vi "Host Matsya 6000.vi"(6 "Channel Data":cluster{"AI":T1, "DI":T5, "DO":T5, "Async":T8}={"AI"={"Interface"="AIO", "Interface Data"={"Command"="Configure", "SubCmd"="AI", "Data"=[{"Channel"="Mod2/ai0", "Min Value"=-5.0, "Max Value"=5.0, "Type"="Voltage", "Terminal Configure"=10083, "Dynamic"=0, "Dyn Type"="", "Data"=[], "File Name"="", "Column"=0, "Frequency"=0.0}, {"Channel"="Mod2/ai1", "Min Value"=-5.0, "Max Value"=5.0, "Type"="Voltage", "Terminal Configure"=10083, "Dynamic"=0, "Dyn Type"="", "Data"=[], "File Name"="", "Column"=0, "Frequency"=0.0}, {"Channel"="Mod2/ai2", "Min Value"=-5.0, "Max Value"=5.0, "Type"="Voltage", "Terminal Configure"=10083, "Dynamic"=0, "Dyn Type"="", "Data"=[], "File Name"="", "Column"=0, "Frequency"=0.0}, {"Channel"="Mod2/ai3", "Min Value"=-5.0, "Max Value"=5.0, "Type"="Voltage", "Terminal Configure"=10083, "Dynamic"=0, "Dyn Type"="", "Data"=[], "File Name"="", "Column"=0, "Frequency"=0.0}, {"Channel"="Mod2/ai4", "Min Value"=-5.0, "Max Value"=5.0, "Type"="Voltage", "Terminal Configure"=10083, "Dynamic"=0, "Dyn Type"="", "Data"=[], "File Name"="", "Column"=0, "Frequency"=0.0}, {"Channel"="Mod2/ai5", "Min Value"=-5.0, "Max Value"=5.0, "Type"="Voltage", "Terminal Configure"=10083, "Dynamic"=0, "Dyn Type"="", "Data"=[], "File Name"="", "Column"=0, "Frequency"=0.0}, {"Channel"="Mod2/ai6", "Min Value"=-5.0, "Max Value"=5.0, "Type"="Voltage", "Terminal Configure"=10083, "Dynamic"=0, "Dyn Type"="", "Data"=[], "File Name"="", "Column"=0, "Frequency"=0.0}, {"Channel"="Mod2/ai7", "Min Value"=-5.0, "Max Value"=5.0, "Type"="Voltage", "Terminal Configure"=10083, "Dynamic"=0, "Dyn Type"="", "Data"=[], "File Name"="", "Column"=0, "Frequency"=0.0}, {"Channel"="Mod2/ai8", "Min Value"=-5.0, "Max Value"=5.0, "Type"="Voltage", "Terminal Configure"=10083, "Dynamic"=0, "Dyn Type"="", "Data"=[], "File Name"="", "Column"=0, "Frequency"=0.0}, {"Channel"="Mod2/ai9", "Min Value"=-5.0, "Max Value"=5.0, "Type"="Voltage", "Terminal Configure"=10083, "Dynamic"=0, "Dyn Type"="", "Data"=[], "File Name"="", "Column"=0, "Frequency"=0.0}, {"Channel"="Mod2/ai10", "Min Value"=-5.0, "Max Value"=5.0, "Type"="Voltage", "Terminal Configure"=10083, "Dynamic"=0, "Dyn Type"="", "Data"=[], "File Name"="", "Column"=0, "Frequency"=0.0}, {"Channel"="Mod2/ai11", "Min Value"=-5.0, "Max Value"=5.0, "Type"="Voltage", "Terminal Configure"=10083, "Dynamic"=0, "Dyn Type"="", "Data"=[], "File Name"="", "Column"=0, "Frequency"=0.0}, {"Channel"="Mod2/ai12", "Min Value"=-5.0, "Max Value"=5.0, "Type"="Voltage", "Terminal Configure"=10083, "Dynamic"=0, "Dyn Type"="", "Data"=[], "File Name"="", "Column"=0, "Frequency"=0.0}, {"Channel"="Mod2/ai13", "Min Value"=-5.0, "Max Value"=5.0, "Type"="Voltage", "Terminal Configure"=10083, "Dynamic"=0, "Dyn Type"="", "Data"=[], "File Name"="", "Column"=0, "Frequency"=0.0}, {"Channel"="Mod2/ai14", "Min Value"=-5.0, "Max Value"=5.0, "Type"="Voltage", "Terminal Configure"=10083, "Dynamic"=0, "Dyn Type"="", "Data"=[], "File Name"="", "Column"=0, "Frequency"=0.0}, {"Channel"="Mod2/ai15", "Min Value"=-5.0, "Max Value"=5.0, "Type"="Voltage", "Terminal Configure"=10083, "Dynamic"=0, "Dyn Type"="", "Data"=[], "File Name"="", "Column"=0, "Frequency"=0.0}, {"Channel"="Mod2/ai16", "Min Value"=-5.0, "Max Value"=5.0, "Type"="Voltage", "Terminal Configure"=10083, "Dynamic"=0, "Dyn Type"="", "Data"=[], "File Name"="", "Column"=0, "Frequency"=0.0}, {"Channel"="Mod2/ai17", "Min Value"=-5.0, "Max Value"=5.0, "Type"="Voltage", "Terminal Configure"=10083, "Dynamic"=0, "Dyn Type"="", "Data"=[], "File Name"="", "Column"=0, "Frequency"=0.0}, {"Channel"="Mod2/ai18", "Min Value"=-5.0, "Max Value"=5.0, "Type"="Voltage", "Terminal Configure"=10083, "Dynamic"=0, "Dyn Type"="", "Data"=[], "File Name"="", "Column"=0, "Frequency"=0.0}, {"Channel"="Mod2/ai19", "Min Value"=-5.0, "Max Value"=5.0, "Type"="Voltage", "Terminal Configure"=10083, "Dynamic"=0, "Dyn Type"="", "Data"=[], "File Name"="", "Column"=0, "Frequency"=0.0}, {"Channel"="Mod2/ai20", "Min Value"=-5.0, "Max Value"=5.0, "Type"="Voltage", "Terminal Configure"=10083, "Dynamic"=0, "Dyn Type"="", "Data"=[], "File Name"="", "Column"=0, "Frequency"=0.0}, {"Channel"="Mod2/ai21", "Min Value"=-5.0, "Max Value"=5.0, "Type"="Voltage", "Terminal Configure"=10083, "Dynamic"=0, "Dyn Type"="", "Data"=[], "File Name"="", "Column"=0, "Frequency"=0.0}, {"Channel"="Mod2/ai22", "Min Value"=-5.0, "Max Value"=5.0, "Type"="Voltage", "Terminal Configure"=10083, "Dynamic"=0, "Dyn Type"="", "Data"=[], "File Name"="", "Column"=0, "Frequency"=0.0}, {"Channel"="Mod2/ai23", "Min Value"=-5.0, "Max Value"=5.0, "Type"="Voltage", "Terminal Configure"=10083, "Dynamic"=0, "Dyn Type"="", "Data"=[], "File Name"="", "Column"=0, "Frequency"=0.0}, {"Channel"="Mod2/ai24", "Min Value"=-5.0, "Max Value"=5.0, "Type"="Voltage", "Terminal Configure"=10083, "Dynamic"=0, "Dyn Type"="", "Data"=[], "File Name"="", "Column"=0, "Frequency"=0.0}, {"Channel"="Mod2/ai25", "Min Value"=-5.0, "Max Value"=5.0, "Type"="Voltage", "Terminal Configure"=10083, "Dynamic"=0, "Dyn Type"="", "Data"=[], "File Name"="", "Column"=0, "Frequency"=0.0}, {"Channel"="Mod2/ai26", "Min Value"=-5.0, "Max Value"=5.0, "Type"="Voltage", "Terminal Configure"=10083, "Dynamic"=0, "Dyn Type"="", "Data"=[], "File Name"="", "Column"=0, "Frequency"=0.0}, {"Channel"="Mod2/ai27", "Min Value"=-5.0, "Max Value"=5.0, "Type"="Voltage", "Terminal Configure"=10083, "Dynamic"=0, "Dyn Type"="", "Data"=[], "File Name"="", "Column"=0, "Frequency"=0.0}, {"Channel"="Mod2/ai28", "Min Value"=-5.0, "Max Value"=5.0, "Type"="Voltage", "Terminal Configure"=10083, "Dynamic"=0, "Dyn Type"="", "Data"=[], "File Name"="", "Column"=0, "Frequency"=0.0}, {"Channel"="Mod2/ai29", "Min Value"=-5.0, "Max Value"=5.0, "Type"="Voltage", "Terminal Configure"=10083, "Dynamic"=0, "Dyn Type"="", "Data"=[], "File Name"="", "Column"=0, "Frequency"=0.0}, {"Channel"="Mod2/ai30", "Min Value"=-5.0, "Max Value"=5.0, "Type"="Voltage", "Terminal Configure"=10083, "Dynamic"=0, "Dyn Type"="", "Data"=[], "File Name"="", "Column"=0, "Frequency"=0.0}, {"Channel"="Mod2/ai31", "Min Value"=-5.0, "Max Value"=5.0, "Type"="Voltage", "Terminal Configure"=65535, "Dynamic"=0, "Dyn Type"="", "Data"=[], "File Name"="", "Column"=0, "Frequency"=0.0}], "Timing"={"samples per channel"=4, "sample mode"=10123, "rate"=2.0}}}, "DI"={"Interface"="DIO", "Interface Data"={"Command"="Configure", "SubCmd"="DI", "Frequency"=500, "Data"=[{"Channel"="Mod3/port0/line0", "Data"=[0], "Identification Name"=""}, {"Channel"="Mod3/port0/line1", "Data"=[0], "Identification Name"=""}, {"Channel"="Mod3/port0/line2", "Data"=[0], "Identification Name"=""}, {"Channel"="Mod3/port0/line3", "Data"=[0], "Identification Name"=""}, {"Channel"="Mod3/port0/line4", "Data"=[0], "Identification Name"=""}, {"Channel"="Mod3/port0/line5", "Data"=[0], "Identification Name"=""}, {"Channel"="Mod3/port0/line6", "Data"=[0], "Identification Name"=""}, {"Channel"="Mod3/port0/line7", "Data"=[0], "Identification Name"=""}, {"Channel"="Mod3/port0/line8", "Data"=[0], "Identification Name"=""}, {"Channel"="Mod3/port0/line9", "Data"=[0], "Identification Name"=""}, {"Channel"="Mod3/port0/line10", "Data"=[0], "Identification Name"=""}, {"Channel"="Mod3/port0/line11", "Data"=[0], "Identification Name"=""}, {"Channel"="Mod3/port0/line12", "Data"=[0], "Identification Name"=""}, {"Channel"="Mod3/port0/line13", "Data"=[0], "Identification Name"=""}, {"Channel"="Mod3/port0/line14", "Data"=[0], "Identification Name"=""}, {"Channel"="Mod3/port0/line15", "Data"=[0], "Identification Name"=""}, {"Channel"="Mod3/port0/line16", "Data"=[0], "Identification Name"=""}, {"Channel"="Mod3/port0/line17", "Data"=[0], "Identification Name"=""}, {"Channel"="Mod3/port0/line18", "Data"=[0], "Identification Name"=""}, {"Channel"="Mod3/port0/line19", "Data"=[0], "Identification Name"=""}, {"Channel"="Mod3/port0/line20", "Data"=[0], "Identification Name"=""}, {"Channel"="Mod3/port0/line21", "Data"=[0], "Identification Name"=""}, {"Channel"="Mod3/port0/line22", "Data"=[0], "Identification Name"=""}, {"Channel"="Mod3/port0/line23", "Data"=[0], "Identification Name"=""}, {"Channel"="Mod3/port0/line24", "Data"=[0], "Identification Name"=""}, {"Channel"="Mod3/port0/line25", "Data"=[0], "Identification Name"=""}, {"Channel"="Mod3/port0/line26", "Data"=[0], "Identification Name"=""}, {"Channel"="Mod3/port0/line27", "Data"=[0], "Identification Name"=""}, {"Channel"="Mod3/port0/line28", "Data"=[0], "Identification Name"=""}, {"Channel"="Mod3/port0/line29", "Data"=[0], "Identification Name"=""}, {"Channel"="Mod3/port0/line30", "Data"=[0], "Identification Name"=""}, {"Channel"="Mod3/port0/line31", "Data"=[0], "Identification Name"=""}, {"Channel"="Mod4/port0/line0", "Data"=[0], "Identification Name"=""}, {"Channel"="Mod4/port0/line1", "Data"=[0], "Identification Name"=""}, {"Channel"="Mod4/port0/line2", "Data"=[0], "Identification Name"=""}, {"Channel"="Mod4/port0/line3", "Data"=[0], "Identification Name"=""}, {"Channel"="Mod4/port0/line4", "Data"=[0], "Identification Name"=""}, {"Channel"="Mod4/port0/line5", "Data"=[0], "Identification Name"=""}, {"Channel"="Mod4/port0/line6", "Data"=[0], "Identification Name"=""}, {"Channel"="Mod4/port0/line7", "Data"=[0], "Identification Name"=""}, {"Channel"="Mod4/port0/line8", "Data"=[0], "Identification Name"=""}, {"Channel"="Mod4/port0/line9", "Data"=[0], "Identification Name"=""}, {"Channel"="Mod4/port0/line10", "Data"=[0], "Identification Name"=""}, {"Channel"="Mod4/port0/line11", "Data"=[0], "Identification Name"=""}, {"Channel"="Mod4/port0/line12", "Data"=[0], "Identification Name"=""}, {"Channel"="Mod4/port0/line13", "Data"=[0], "Identification Name"=""}, {"Channel"="Mod4/port0/line14", "Data"=[0], "Identification Name"=""}, {"Channel"="Mod4/port0/line15", "Data"=[0], "Identification Name"=""}, {"Channel"="Mod4/port0/line16", "Data"=[0], "Identification Name"=""}, {"Channel"="Mod4/port0/line17", "Data"=[0], "Identification Name"=""}, {"Channel"="Mod4/port0/line18", "Data"=[0], "Identification Name"=""}, {"Channel"="Mod4/port0/line19", "Data"=[0], "Identification Name"=""}, {"Channel"="Mod4/port0/line20", "Data"=[0], "Identification Name"=""}, {"Channel"="Mod4/port0/line21", "Data"=[0], "Identification Name"=""}, {"Channel"="Mod4/port0/line22", "Data"=[0], "Identification Name"=""}, {"Channel"="Mod4/port0/line23", "Data"=[0], "Identification Name"=""}, {"Channel"="Mod4/port0/line24", "Data"=[0], "Identification Name"=""}, {"Channel"="Mod4/port0/line25", "Data"=[0], "Identification Name"=""}, {"Channel"="Mod4/port0/line26", "Data"=[0], "Identification Name"=""}, {"Channel"="Mod4/port0/line27", "Data"=[0], "Identification Name"=""}, {"Channel"="Mod4/port0/line28", "Data"=[0], "Identification Name"=""}, {"Channel"="Mod4/port0/line29", "Data"=[0], "Identification Name"=""}, {"Channel"="Mod4/port0/line30", "Data"=[0], "Identification Name"=""}, {"Channel"="Mod4/port0/line31", "Data"=[0], "Identification Name"=""}]}}, "DO"={"Interface"="DIO", "Interface Data"={"Command"="Configure", "SubCmd"="DO", "Frequency"=500, "Data"=[{"Channel"="Mod1/port0/line0", "Data"=[0], "Identification Name"=""}, {"Channel"="Mod1/port0/line1", "Data"=[0], "Identification Name"=""}, {"Channel"="Mod1/port0/line2", "Data"=[0], "Identification Name"=""}, {"Channel"="Mod1/port0/line3", "Data"=[0], "Identification Name"=""}, {"Channel"="Mod1/port0/line4", "Data"=[0], "Identification Name"=""}, {"Channel"="Mod1/port0/line5", "Data"=[0], "Identification Name"=""}, {"Channel"="Mod1/port0/line6", "Data"=[0], "Identification Name"=""}, {"Channel"="Mod1/port0/line7", "Data"=[0], "Identification Name"=""}, {"Channel"="Mod1/port0/line8", "Data"=[0], "Identification Name"=""}, {"Channel"="Mod1/port0/line9", "Data"=[0], "Identification Name"=""}, {"Channel"="Mod1/port0/line10", "Data"=[0], "Identification Name"=""}, {"Channel"="Mod1/port0/line11", "Data"=[0], "Identification Name"=""}, {"Channel"="Mod1/port0/line12", "Data"=[0], "Identification Name"=""}, {"Channel"="Mod1/port0/line13", "Data"=[0], "Identification Name"=""}, {"Channel"="Mod1/port0/line14", "Data"=[0], "Identification Name"=""}, {"Channel"="Mod1/port0/line15", "Data"=[0], "Identification Name"=""}, {"Channel"="Mod1/port0/line16", "Data"=[0], "Identification Name"=""}, {"Channel"="Mod1/port0/line17", "Data"=[0], "Identification Name"=""}, {"Channel"="Mod1/port0/line18", "Data"=[0], "Identification Name"=""}, {"Channel"="Mod1/port0/line19", "Data"=[0], "Identification Name"=""}, {"Channel"="Mod1/port0/line20", "Data"=[0], "Identification Name"=""}, {"Channel"="Mod1/port0/line21", "Data"=[0], "Identification Name"=""}, {"Channel"="Mod1/port0/line22", "Data"=[0], "Identification Name"=""}, {"Channel"="Mod1/port0/line23", "Data"=[0], "Identification Name"=""}, {"Channel"="Mod1/port0/line24", "Data"=[0], "Identification Name"=""}, {"Channel"="Mod1/port0/line25", "Data"=[0], "Identification Name"=""}, {"Channel"="Mod1/port0/line26", "Data"=[0], "Identification Name"=""}, {"Channel"="Mod1/port0/line27", "Data"=[0], "Identification Name"=""}, {"Channel"="Mod1/port0/line28", "Data"=[0], "Identification Name"=""}, {"Channel"="Mod1/port0/line29", "Data"=[0], "Identification Name"=""}, {"Channel"="Mod1/port0/line30", "Data"=[0], "Identification Name"=""}, {"Channel"="Mod1/port0/line31", "Data"=[0], "Identification Name"=""}]}}, "Async"={"Interface"="Async", "Interface Data"={"Command"="Configure", "SubCmd"="Async", "Data"=[{"Port"="com10", "Minor Frame Freq"=200, "Minor Frame Count"=1, "Frame Info"=[{"Frame ID"=1, "Message Info"=[{"Message"=[1], "Message Name"="m1"}]}], "Sensor Type"=0, "OIM Address"=0}]}}} {"Async"."Interface Data"."Data"."Minor Frame Count" min=5 max=8 step=1; "AI"."Interface Data"."Timing"."sample mode" items=["Finite Samples"=10178, "Continuous Samples"=10123, "Hardware Timed Single Point"=12522]}, 11 "address":string="192.168.81.153") -> ()   [LabVIEW 2021]
uses:
  Main Engine/Controls/Main Engine CPU Info.ctl
  Host/Controls/Host Data Cluster.ctl
  Async Serial/Controls/Async Update Cluster.ctl
  Async Serial/Controls/Async Message Info Cluster.ctl
  Analog Output/Controls/AO Timing Cluster.ctl
  Analog Output/Controls/AO Channel Configuration Cluster.ctl
  Analog Output/Controls/AO Interface Data Cluster.ctl
  Analog Output/Controls/AO JSON Data Cluster.ctl
  Digital Output/SubVIs/Digital Dynamic Cluster.ctl
  Digital Output/Controls/DIO Interface Data.ctl
  Digital Output/Controls/DIO Configuration cluster.ctl
  Async Serial/Controls/Async Frame Info Cluster.ctl
  Async Serial/Controls/Async Serial Configuration Cluster.ctl
  Host/Async Interface Data Cluster.ctl
  Host/Async JSON Cluster.ctl
panel:
  out "error out 3":errorcluster
  out "error out 2":errorcluster
  out "Data Out":T13
  out "Stop":bool
  out "error out":errorcluster
  in  "Tab Control":T15(tab)
  in  "Send DIO Update":bool
  in  "DO Data":cluster{"Channel":string[], "Data":u8[]}={"Channel"=["Mod2/port1/line0", "Mod2/port1/line1", "Mod2/port1/line2", "Mod2/port1/line3"], "Data"=[0, 0, 0, 0]}
  in  "Send Async Update":bool
  in  "Serial Data":T16[](array[typedef])
  in  "Async Stop":string="{\"Interface\":\"Async\",\"Interface Data\":{\"Command\":\"Stop\",\"SubCmd\":\"Async\",\"Data\":[\"com2\"]}}"
  in  "Send Async Stop":bool
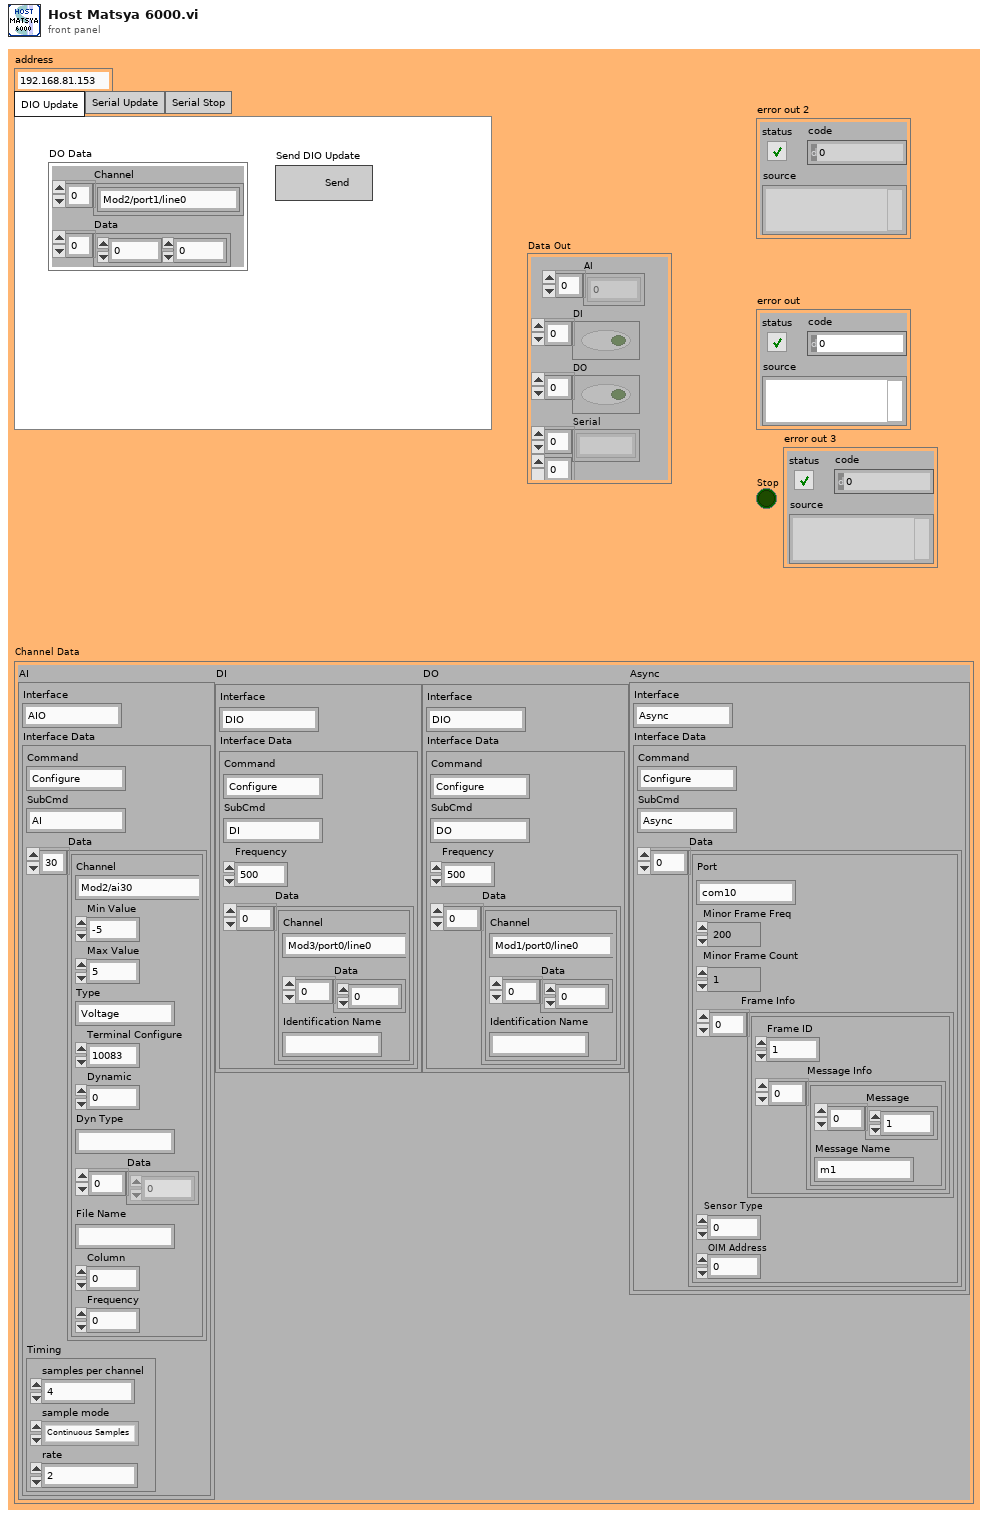
[diagram p1: front panel]
types:
  T1 = typedef "AO JSON Data Cluster.ctl" = cluster{"Interface":string, "Interface Data":T2}
  T2 = typedef "AO Interface Data Cluster.ctl" = cluster{"Command":string, "SubCmd":string, "Data":T3[], "Timing":T4}
  T3 = typedef "AO Channel Configuration Cluster.ctl" = cluster{"Channel":string, "Min Value":dbl, "Max Value":dbl, "Type":string, "Terminal Configure":u16, "Dynamic":u8, "Dyn Type":string, "Data":dbl[], "File Name":string, "Column":i32, "Frequency":dbl}
  T4 = typedef "AO Timing Cluster.ctl" = cluster{"samples per channel":i32, "sample mode":i32, "rate":dbl}
  T5 = typedef "DIO Configuration cluster.ctl" = cluster{"Interface":string, "Interface Data":T6}
  T6 = typedef "DIO Interface Data.ctl" = cluster{"Command":string, "SubCmd":string, "Frequency":u16, "Data":T7[]}
  T7 = typedef "Digital Dynamic Cluster.ctl" = cluster{"Channel":string, "Data":u8[], "Identification Name":string}
  T8 = typedef "Async JSON Cluster.ctl" = cluster{"Interface":string, "Interface Data":T9}
  T9 = typedef "Async Interface Data Cluster.ctl" = cluster{"Command":string, "SubCmd":string, "Data":T10[]}
  T10 = typedef "Async Serial Configuration Cluster.ctl" = cluster{"Port":string, "Minor Frame Freq":u16, "Minor Frame Count":u16, "Frame Info":T11[], "Sensor Type":u16, "OIM Address":u16}
  T11 = typedef "Async Frame Info Cluster.ctl" = cluster{"Frame ID":u16, "Message Info":T12[]}
  T12 = typedef "Async Message Info Cluster.ctl" = cluster{"Message":u8[], "Message Name":string}
  T13 = typedef "Host Data Cluster.ctl" = cluster{"AI":dbl[], "DI":bool[], "DO":bool[], "Serial":string[][], "CPU":T14, "Stop":bool, "DO Channel":string[]}
  T14 = typedef "Main Engine CPU Info.ctl" = cluster{"Total Load":u32[], "Interrupt Load":u32[], "Total Physical":dbl, "Free Physical":dbl, "Primary Disk Capacity":dbl, "Primary Disk Free":dbl}
  T15 = enum32{"DIO Update", "DIO stop", "Serial Update", "Serial Stop"}
  T16 = typedef "Async Update Cluster.ctl" = cluster{"Port":string, "Message Info":T12[]}
  T17 = enum16{"Initialize", "Read", "Update DO", "Update Serial", "Exit"}
  T18 = enum16{"big-endian, network order", "native, host order", "little-endian"}
  T19 = typedef "RT Data's.ctl" = cluster{"RT HW Info":T20, "DO Info":T24}
  T20 = typedef "RT HW Info.ctl" = cluster{"Serial Hardware Info JSON Format":T21, "Analog HW Info JSON Format":T22, "Digital HW Info JSON Format":T22, "Ethernet IP Address JSON Format":T23}
  T21 = typedef "Main Engine Serial Info JSON Data.ctl" = cluster{"Command":string, "SubCmd":string, "Channel":string[]}
  T22 = typedef "Main Engine DAQ Harware Info JSON Data.ctl" = cluster{"Command":string, "SubCmd":string, "Input":string[], "Output":string[]}
  T23 = typedef "Main Engine Ehernet IP Address JSON Data.ctl" = cluster{"Command":string, "SubCmd":string, "IP":string[]}
  T24 = typedef "DIO Data's from RT.ctl" = cluster{"Channels":string[], "Data":bool[], "Time":string}
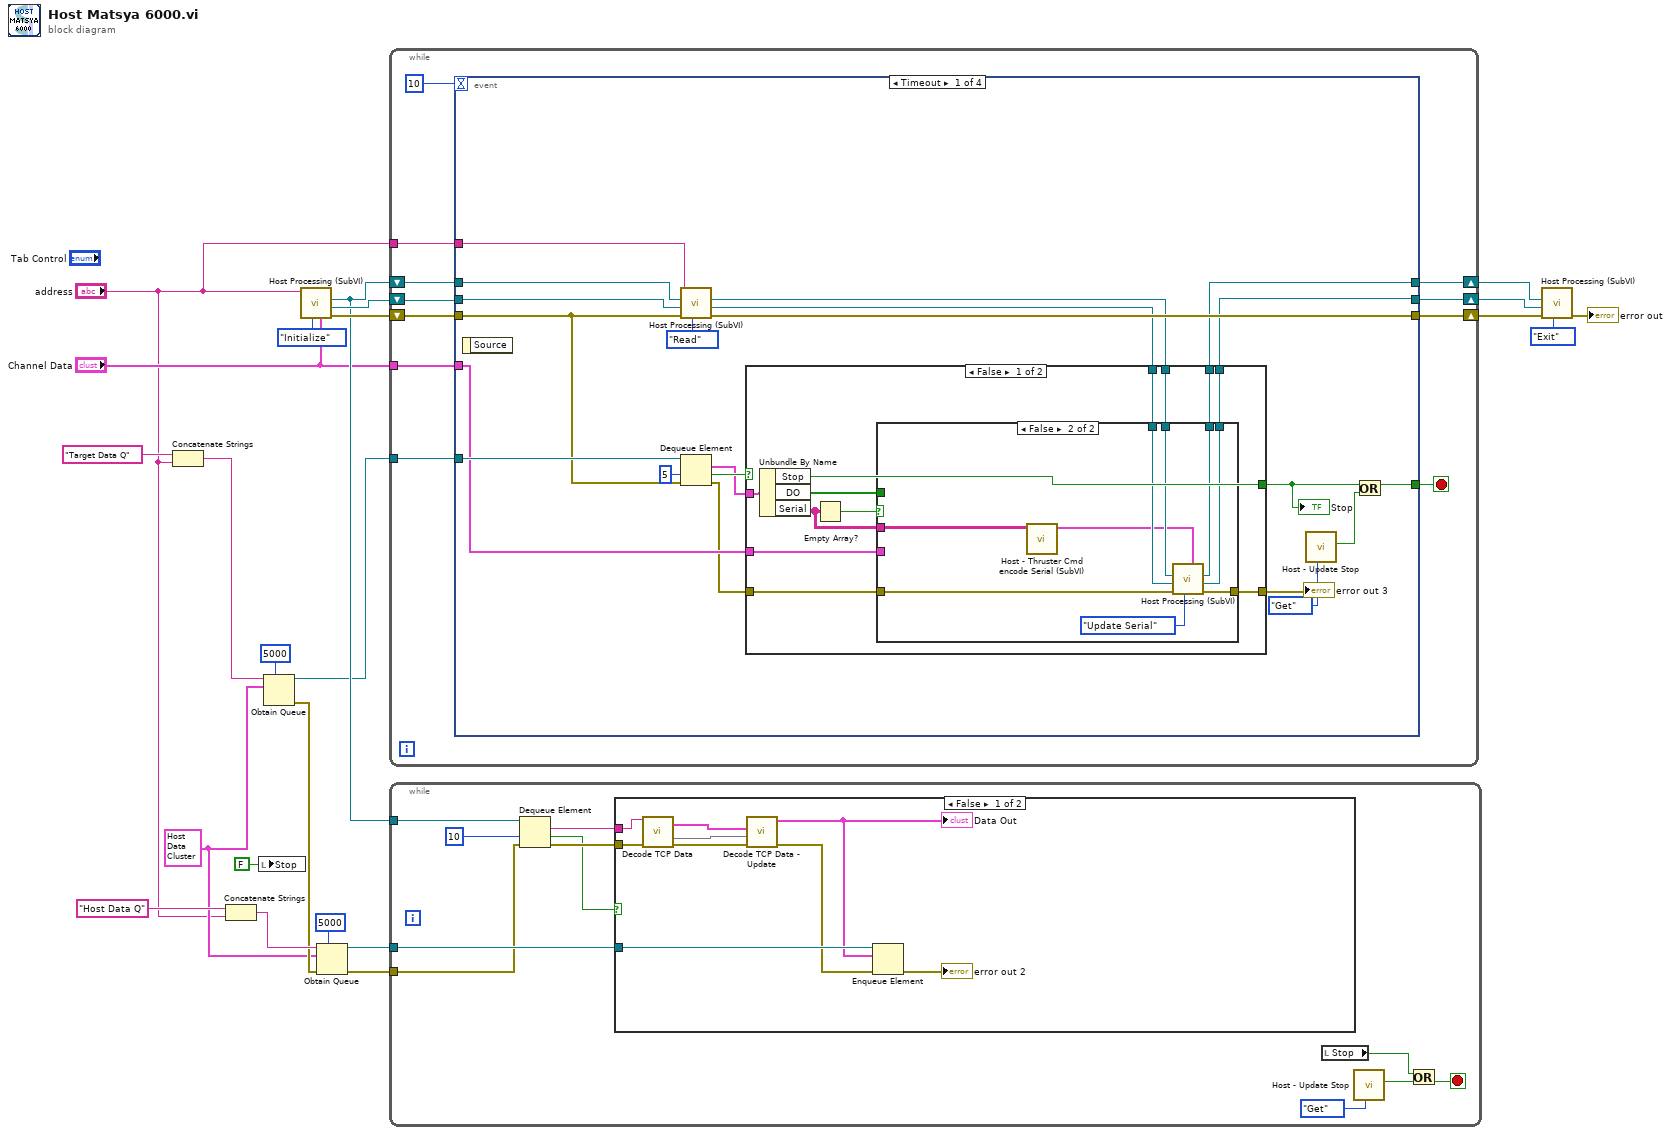
[diagram p0: block diagram]
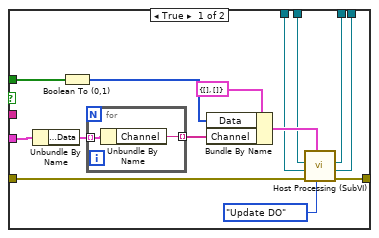
[diagram p3: hidden frame]
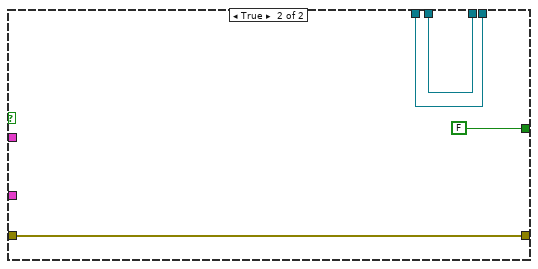
[diagram p4: hidden frame]
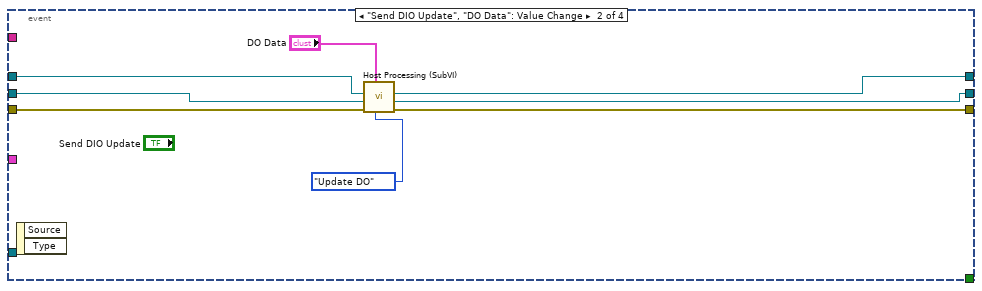
[diagram p5: hidden frame]
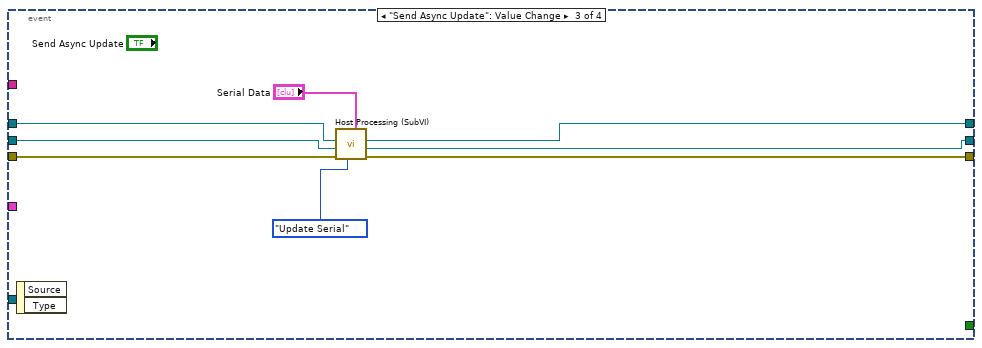
[diagram p6: hidden frame]
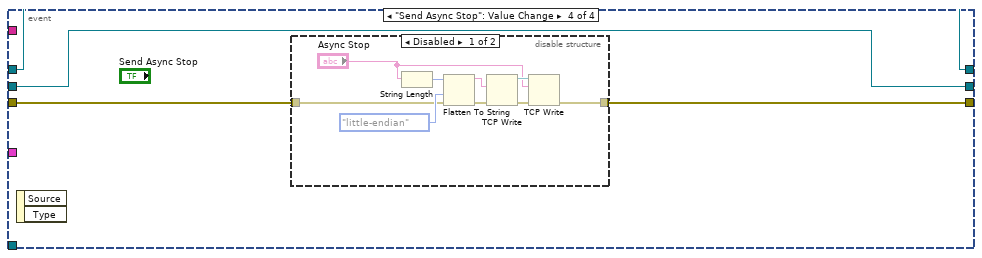
[diagram p7: hidden frame]
diagram:
  w4 = T13 {"AI"=[-3.29963760152739, -3.28042607250678, -3.30275742266883, -3.28305329003257, -3.29914499819412, -3.27566424083626, -3.29520417157553, -3.26269235518028, -3.14446761533159, -3.13215254239399, -3.16088771377303, -3.13198834142664, -3.16959036650255, -3.151528257494, -3.17188918049567, -3.1431540075152, -3.2208210848143, -3.21425304324317, -3.24479443847459, -3.23132995179905, -3.24922786722435, -3.22706072451644, -3.22311989941762, -3.18896608529332, -3.07895143597999, -3.07616002028715, -3.11064221681751, -3.08551947305428, -3.12459929803547, -3.10916440827463, -3.12197208267327], "DI"=[FALSE, FALSE, FALSE, FALSE, FALSE, FALSE, FALSE, FALSE, FALSE, FALSE, FALSE, FALSE, FALSE, FALSE, FALSE, FALSE, FALSE, FALSE, FALSE, FALSE, FALSE, FALSE, FALSE, FALSE, FALSE, FALSE, FALSE, FALSE, FALSE, FALSE, FALSE, FALSE, FALSE, FALSE, FALSE, FALSE, FALSE, FALSE, FALSE, FALSE, FALSE, FALSE, FALSE, FALSE, FALSE, FALSE, FALSE, FALSE, FALSE, FALSE, FALSE, FALSE, FALSE, FALSE, FALSE, FALSE, FALSE, FALSE, FALSE, FALSE, FALSE, FALSE, FALSE, FALSE], "DO"=[], "Serial"=[], "CPU"={"Total Load"=[], "Interrupt Load"=[], "Total Physical"=0.0, "Free Physical"=0.0, "Primary Disk Capacity"=0.0, "Primary Disk Free"=0.0}, "Stop"=FALSE, "DO Channel"=[]} ("Data Out")
  n1 = Concatenate Strings("Target Data Q" ("name (unnamed)"), "address") -> (w7:string)
  n2 = Concatenate Strings("Host Data Q" ("name (unnamed)"), "address") -> (w22:string)
  n3 = local write "Stop"(FALSE ("Stop")) -> ()
  n4 = Obtain Queue(max queue size (-1, unlimited)=5000, name (unnamed)=w7, element data type=w4) -> (queue out=w3:refnum<queue>, error out=w5:errorcluster)  [unwired: 2 in, 1 out]
  n5 = call "Host Processing (SubVI).vi"("Channel Data"="Channel Data", "Operation"=T17."Initialize", "IP"="address") -> ("error out"=w16:errorcluster, "connection ID"=w12:refnum<k5>, "Queue out"=w11:refnum<queue>)  [unwired: 5 in, 1 out]
  n6 = Obtain Queue(max queue size (-1, unlimited)=5000, name (unnamed)=w22, element data type=w4, error in (no error)=w5) -> (queue out=w19:refnum<queue>, error out=w18:errorcluster)  [unwired: 1 in, 1 out]
  n7 = while {
    shift-right: [w32] -> w15
    shift-left: w16 -> [w34]
    shift-right: [w28] -> w9
    shift-left: w11 -> [w30]
    shift-right: [w27] -> w10
    shift-left: w12 -> [w29]
    tunnel: w3 -> [w26]
    tunnel: "Channel Data" -> [w25]
    tunnel: "address" -> [w24]
    stop <- w33 stop-if-true
    n8 = event shown="[0] Timeout" {
      selector: _ -> [_ _ _ _]
      dyn-events: _ -> [_ _ _ _]
      timeout: 10 -> [_ _ _ _]
      tunnel: w34 -> [w47 w104 w111 w116]
      tunnel: [w38 _ _ _] -> w33
      tunnel: [w54 w101 w110 w115] -> w32
      tunnel: w30 -> [w52 w100 w108 w114]
      tunnel: w29 -> [w53 w99 w107 w113]
      tunnel: [w41 w98 w106 w114] -> w28
      tunnel: [w39 w97 w105 w113] -> w27
      tunnel: w26 -> [w49 _ _ _]
      tunnel: w25 -> [w48 _ _ _]
      tunnel: w24 -> [w36 _ _ _]
      event Timeout {
        n9 = event-data() -> ()  [unwired: 1 in, 1 out]
        n10 = call "Host Processing (SubVI).vi"("Operation"=T17."Read", "error in"=w47, "connection ID in"=w53, "queue in"=w52, "IP"=w36) -> ("error out"=w54:errorcluster, "connection ID"=w40:refnum<k5>, "Queue out"=w42:refnum<queue>)  [unwired: 3 in, 1 out]
        n11 = Dequeue Element(queue=w49, timeout in ms (-1)=5, error in (no error)=w47) -> (element=w50:T13, timed out?=w51:bool, error out=w46:errorcluster)  [unwired: 1 out]
        n12 = case shown="False" w51 {
          tunnel: w50 -> [w67 _]
          tunnel: w48 -> [w66 _]
          tunnel: [w64 FALSE ("Stop")] -> w44
          tunnel: w46 -> [w63 w95]
          tunnel: [w62 w95] -> w45
          tunnel: w42 -> [w61 w94]
          tunnel: [w60 w94] -> w41
          tunnel: w40 -> [w59 w93]
          tunnel: [w58 w93] -> w39
          frame False {
            n13 = Unbundle By Name(w67) -> ("Stop"=w64:bool, "DO"=w65:bool[], "Serial"=w56:string[][])
            n14 = Empty Array?(array=w56) -> (empty?=w57:bool)
            n15 = case shown="False" w57 {
              tunnel: w66 -> [w81 _]
              tunnel: w65 -> [w78 _]
              tunnel: w63 -> [w73 w91]
              tunnel: [w72 w90] -> w62
              tunnel: w61 -> [w71 w89]
              tunnel: [w70 w88] -> w60
              tunnel: w59 -> [w69 w87]
              tunnel: [w68 w86] -> w58
              tunnel: w56 -> [_ w84]
              frame True {
                n16 = Unbundle By Name(w81) -> ("DO.Interface Data.Data"=w80:T7[])
                n17 = Boolean To (0,1)(Boolean=w78) -> (0, 1=w77:i16[])
                n18 = for {
                  tunnel: w80 -> [w83] mode=indexing
                  tunnel: [w82] -> w76 mode=indexing
                  n19 = Unbundle By Name(w83) -> ("Channel"=w82:string)
                }
                n20 = Bundle By Name(cluster=cluster{"Channel":string[], "Data":u8[]} {"Channel"=[], "Data"=[]} ("DO Data"), "Data"=w77, "Channel"=w76) -> (w74:cluster{"Channel":string[], "Data":u8[]})
                n21 = call "Host Processing (SubVI).vi"("Operation"=T17."Update DO", "DO Data"=w74, "error in"=w73, "connection ID in"=w69, "queue in"=w71) -> ("error out"=w72:errorcluster, "connection ID"=w68:refnum<k5>, "Queue out"=w70:refnum<queue>)  [unwired: 3 in, 1 out]
              }
              frame False {
                n22 = call "Host - Thruster Cmd encode Serial (SubVI).vi"("Serial"=w84) -> ("Serial Data"=w85:T16[])  [unwired: 10 in]
                n23 = call "Host Processing (SubVI).vi"("Serial Data"=w85, "Operation"=T17."Update Serial", "error in"=w91, "connection ID in"=w87, "queue in"=w89) -> ("error out"=w90:errorcluster, "connection ID"=w86:refnum<k5>, "Queue out"=w88:refnum<queue>)  [unwired: 3 in, 1 out]
              }
            }
          }
          frame True {
          }
        }
        "error out 3" <- w45
        "Stop" <- w44
        n24 = call "Host - Update Stop.vi"("Operation"=enum16{"Init", "Get", "Set"}."Get") -> ("Stop?"=w37:bool)  [unwired: 9 in, 1 out]
        n25 = Or(x=w44, y=w37) -> (x .or. y?=w38:bool)
      }
      event "Send DIO Update", "DO Data": Value Change {
        n26 = event-data() -> ()  [unwired: 1 in, 2 out]
        n27 = call "Host Processing (SubVI).vi"("Operation"=T17."Update DO", "DO Data"="DO Data", "error in"=w104, "connection ID in"=w99, "queue in"=w100) -> ("error out"=w101:errorcluster, "connection ID"=w97:refnum<k5>, "Queue out"=w98:refnum<queue>)  [unwired: 3 in, 1 out]
      }
      event "Send Async Update": Value Change {
        n28 = event-data() -> ()  [unwired: 1 in, 2 out]
        n29 = call "Host Processing (SubVI).vi"("Serial Data"="Serial Data", "Operation"=T17."Update Serial", "error in"=w111, "connection ID in"=w107, "queue in"=w108) -> ("error out"=w110:errorcluster, "connection ID"=w105:refnum<k5>, "Queue out"=w106:refnum<queue>)  [unwired: 3 in, 1 out]
      }
      event "Send Async Stop": Value Change {
        n30 = event-data() -> ()  [unwired: 1 in, 2 out]
        n31 = disable-structure shown="Disabled" {
          disable-tunnel: w116 -> [w119 w126]
          disable-tunnel: [w118 w126] -> w115
          frame Disabled {
            n32 = String Length(string="Async Stop") -> (length=w123:i32)
            n33 = Flatten To String(anything=w123, byte order (0:big-endian, network order)=T18."little-endian", error in (no error)=w119) -> (data string=w121:string, error out=w120:errorcluster)  [unwired: 1 in, 1 out]
            n34 = TCP Write(data in=w121, error in (no error)=w120) -> (connection ID out=w125:refnum<k5>, error out=w124:errorcluster)  [unwired: 2 in, 1 out]
            n35 = TCP Write(connection ID=w125, data in="Async Stop", error in (no error)=w124) -> (error out=w118:errorcluster)  [unwired: 1 in, 2 out]
          }
          frame Enabled {
          }
        }
      }
    }
  }
  n36 = while {
    tunnel: w11 -> [w136]
    tunnel: w19 -> [w137]
    tunnel: w18 -> [w132]
    stop <- w129 stop-if-true
    n37 = Dequeue Element(queue=w136, timeout in ms (-1)=10, error in (no error)=w132) -> (element=w135:string, timed out?=w131:bool, error out=w134:errorcluster)  [unwired: 1 out]
    n38 = case shown="False" w131 {
      tunnel: w137 -> [w146 _]
      tunnel: w135 -> [w145 _]
      tunnel: w134 -> [w141 _]
      frame False {
        n39 = call "Decode TCP Data.vi"("TCP Rx-Tx Cluster In"=w145, "error in"=w141) -> ("RT-Data's Out"=w144:T19, 10:w143, "error out"=w142:errorcluster)  [unwired: 11 in]
        n40 = call "Decode TCP Data - Update.vi"("error in"=w142, "Type"=w143, "Input Data"=w144) -> ("error out"=w140:errorcluster, "Data Out"=w138:T13)  [unwired: 7 in]
        "Data Out" <- w138
        n41 = Enqueue Element(queue=w146, element=w138, error in (no error)=w140) -> (error out=→"error out 2":errorcluster)  [unwired: 1 in, 2 out]
      }
      frame True {
      }
    }
    n42 = local read "Stop"() -> (w128:bool)
    n43 = call "Host - Update Stop.vi"("Operation"=enum16{"Init", "Get", "Set"}."Get") -> ("Stop?"=w130:bool)  [unwired: 9 in, 1 out]
    n44 = Or(x=w128, y=w130) -> (x .or. y?=w129:bool)
  }
  n45 = call "Host Processing (SubVI).vi"("Operation"=T17."Exit", "error in"=w15, "connection ID in"=w10, "queue in"=w9) -> ("error out"=→"error out":errorcluster)  [unwired: 4 in, 3 out]
